vi "Release Module Semaphore.vi"(8 "error in":errorcluster) -> (0 "error out":errorcluster)   [LabVIEW 2017, in "DQMH Power Requests.lvlib"]
doc: "Release the module semaphore.\n_____\nCreated using DQMH Event Scripter 7.0.0.1280."
uses:
  DQMH Power Requests.lvlib
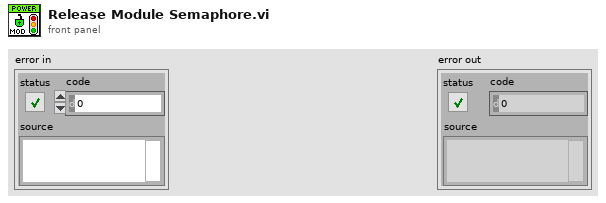
[diagram p1: front panel]
types:
  T1 = typedef "Semaphore RefNum" = refnum<k1>
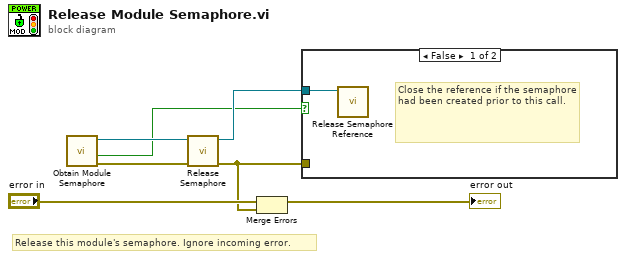
[diagram p0: block diagram]
diagram:
  # "Release this module's semaphore. Ignore incoming error."
  n1 = call "Obtain Module Semaphore.vi"() -> ("error out"=w6:errorcluster, "created new"=w1:bool, "semaphore"=w7:T1)  [unwired: 9 in]
  n2 = call <vilib>:"Release Semaphore.vi"("error in (no error)"=w6, "semaphore"=w7) -> ("error out"=w3:errorcluster, "semaphore out"=w2:T1)  [unwired: 4 in]
  n3 = Merge Errors("error in", w3) -> (→"error out":errorcluster)
  n4 = case shown="False" w1 {
    tunnel: w3 -> [_ _]
    tunnel: w2 -> [w8 _]
    frame False {
      # "Close the reference if the semaphore had been created prior to this call."
      n5 = call <vilib>:"Release Semaphore Reference.vi"("semaphore"=w8) -> ()  [unwired: 9 in, 2 out]
    }
    frame True {
    }
  }
